vi "Delete Registration Code.vi"(8 "error in (no error)":errorcluster, 11 "IoT Session in":refnum<class "IoT Session.lvclass">) -> (0 "error out":errorcluster, 3 "IoT Session out":refnum<class "IoT Session.lvclass">)   [LabVIEW 2015, in "NI_AWS_IoT.lvlib" / "IoT Session.lvclass"]
uses:
  IoT Session.lvclass
  Core/HTTP Request/Request Options.ctl
  Core/HTTP Request/Name Value Pair.ctl
  Core/HTTP Request/Region handling.ctl
  Core/HTTP Request/URL formatting.ctl
  Core/HTTP Request/HTTP Request.lvclass
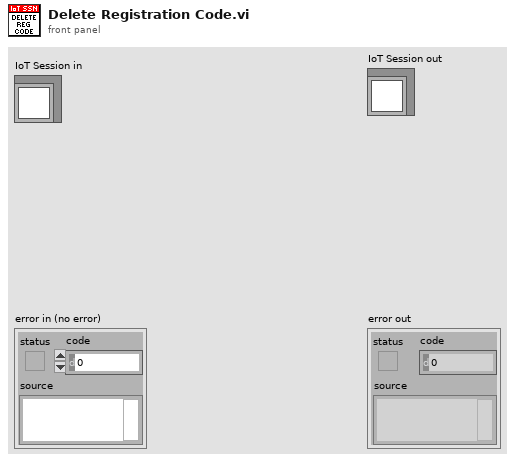
[diagram p1: front panel]
types:
  T1 = typedef "NI_AWS_Core.lvlib/HTTP Request.lvclass/Name Value Pair.ctl" = cluster{"name":string, "value":string}
  T2 = typedef "NI_AWS_Core.lvlib/HTTP Request.lvclass/Request Options.ctl" = cluster{"request headers":T1[], "request parameters":T1[], "request body":string, "region handling":T3, "URL formatting":T4}
  T3 = typedef "NI_AWS_Core.lvlib/HTTP Request.lvclass/Region handling.ctl" = enum16{"use region everywhere", "use region (authentication only)", "use region (URL only)", "ignore region everwhere"}
  T4 = typedef "NI_AWS_Core.lvlib/HTTP Request.lvclass/URL formatting.ctl" = enum16{"region-", "region."}
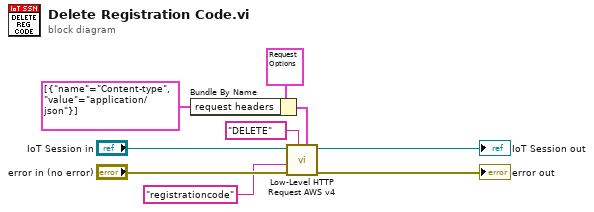
[diagram p0: block diagram]
diagram:
  n1 = Bundle By Name(cluster=T2 {"request headers"=[], "request parameters"=[], "request body"="", "region handling"=enum."use region everywhere", "URL formatting"=enum."region."} ("Request Options"), "request headers"=T1[] [{"name"="Content-type", "value"="application/json"}]) -> (w3:T2)
  n2 = call "Low-Level HTTP Request AWS v4.vi"("Request Options"=w3, "HTTP-Verb"="DELETE", "error in (no error)"="error in (no error)", "URL Suffix"="registrationcode", "AWS Core in"="IoT Session in") -> ("error out"=→"error out":errorcluster, "AWS Core out"=→"IoT Session out":refnum<class "IoT Session.lvclass">)  [unwired: 3 in, 2 out]
